vi "ExposeBoundControlValueChangeCallbackVI.vi"(4 "Expose Info":T1, 6 "CtlRef":refnum<vi>, 7 "Event Common Data":cluster{"Source":T2, "Type":T3, "Time":u32} {"Source" items=["LabVIEW UI"=0, "ActiveX"=1, "User Event"=25]}) -> ()   [LabVIEW 2017]
uses:
  <vilib>/event_ctls.llb/eventsource.ctl
  <vilib>/event_ctls.llb/lveventtype.ctl
  Core/ExposeInfo.ctl
  C:/Code/CMCryoSysCode/Expose/COM/CSCom/CSCom/bin/Release/CSCom.dll
  COM/CSCom/CSCom/bin/Release/CSCom.dll
  ExposeParameterBindingData.ctl
  ExposeParameterBindingType.ctl
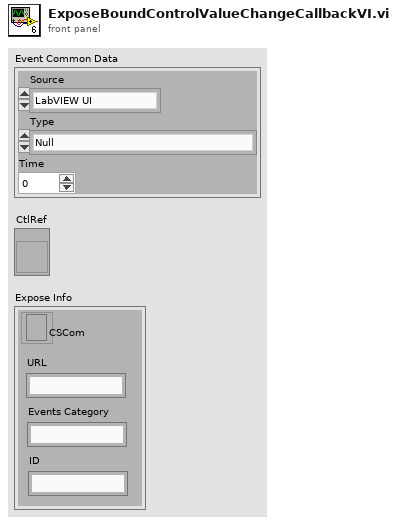
[diagram p1: front panel]
types:
  T1 = typedef "ExposeInfo.ctl" = cluster{"CSCom":refnum<k24>, "URL":string, "Events Category":string, "ID":string}
  T2 = typedef "eventsource.ctl" = u32
  T3 = typedef "lveventtype.ctl" = enum32{"Null", "Timeout", "Annotation Menu Selection", "Annotation Menu Selection?", "App Instance Close", "App Instance Close?", "Autoscale Range Change", "Bookmark Info Change", "Cell Edit", "Cell Edit?", "Cursor Grab", "Cursor Grab?", "Cursor Menu Selection", "Cursor Menu Selection?", "Cursor Move", "Cursor Release", "Data Change", "Direction Change", "Display State Change", "Drag Ended", "Drag Enter", "Drag Leave", "Drag Over", "Drag Source Update", "Drag Starting", "Drag Starting?", "Drop", "Exec State Change", "Key Down", "Key Down?", "Key Repeat", "Key Repeat?", "Key Up", "Listbox Double Click", "Menu Activation?", "Menu Selection (App)", "Menu Selection? (App)", "Menu Selection (User)", "Mouse Down", "Mouse Down?", "Mouse Enter", "Mouse Leave", "Mouse Move", "Mouse Up", "Mouse Wheel", "NI Security User Change (App)", "Pane Size", "Panel Close", "Panel Close?", "Panel Resize", "Plot Attribute Change", "Scale Range Change", "Shortcut Menu Activation?", "Shortcut Menu Selection (App)", "Shortcut Menu Selection? (App)", "Shortcut Menu Selection (User)", "Tree Double Click", "Tree Drag", "Tree Drag?", "Tree Drop", "Tree Drop?", "Tree Item Close", "Tree Item Close?", "Tree Item Open", "Tree Item Open?", "User Event", "Value Change"}
  T4 = typedef "ExposeDataType.ctl" = cluster{"Values":variant, "ParameterBindingInfo":variant}
  T5 = typedef "ExposeParameterBindingData.ctl" = cluster{"Val Change EV":refnum<k27>, "Bind Direction":T6, "Ignore Next\nUpdate Count":i32}
  T6 = typedef "ExposeParameterBindingType.ctl" = enum16{"ToRemote", "FromRemote", "Bidrectional"}
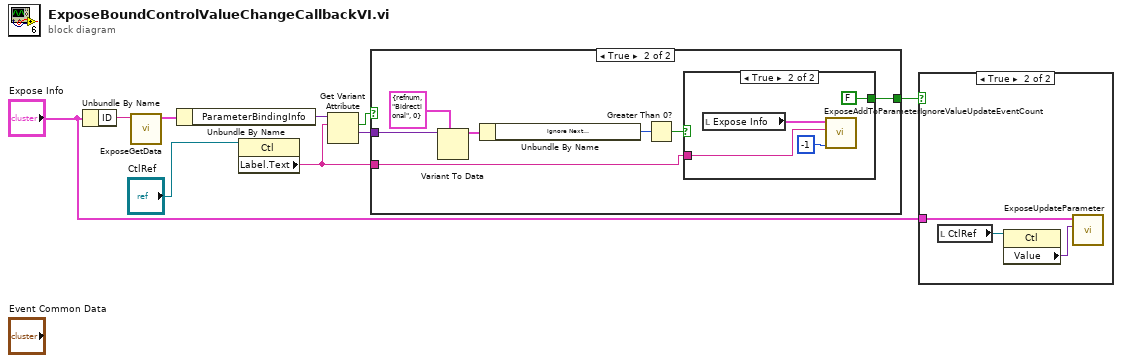
[diagram p0: block diagram]
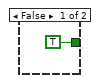
[diagram p3: hidden frame]
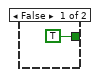
[diagram p4: hidden frame]
diagram:
  n1 = Unbundle By Name("Expose Info") -> ("ID"=w7:string)
  n2 = call "ExposeGetData.vi"("ExposeID"=w7) -> ("ExposeDataType"=w6:T4)  [unwired: 9 in, 1 out]
  n3 = Unbundle By Name(w6) -> ("ParameterBindingInfo"=w5:variant)
  n4 = property class="Ctl"(reference="CtlRef") -> ("Label.Text"=w2:string)  [unwired: 1 in, 2 out]
  n5 = Get Variant Attribute(Variant=w5, name=w2) -> (found=w4:bool, value=w1:variant)  [unwired: 2 in, 2 out]
  n6 = case shown="True" w4 {
    tunnel: [TRUE w13] -> w3
    tunnel: w2 -> [_ w12]
    tunnel: w1 -> [_ w11]
    frame False {
    }
    frame True {
      n7 = Variant To Data(type=T5 {"Val Change EV"=refnum, "Bind Direction"=enum."Bidrectional", "Ignore Next\nUpdate Count"=0} ("ExposeParmeterBindingData"), Variant=w11) -> (data=w16:T5)  [unwired: 1 in, 1 out]
      n8 = Unbundle By Name(w16) -> ("Ignore Next\nUpdate Count"=w15:i32)
      n9 = Greater Than 0?(x=w15) -> (x > 0?=w14:bool)
      n10 = case shown="True" w14 {
        tunnel: [TRUE FALSE] -> w13
        tunnel: w12 -> [_ w20]
        frame False {
        }
        frame True {
          n11 = local read "Expose Info"() -> (w21:T1)
          n12 = call "ExposeAddToParameterIgnoreValueUpdateEventCount.vi"("Add to count (0)"=-1, "Name"=w20, "Expose Info"=w21) -> ()  [unwired: 8 in, 1 out]
        }
      }
    }
  }
  n13 = case shown="True" w3 {
    tunnel: "Expose Info" -> [_ w25]
    frame False {
    }
    frame True {
      n14 = local read "CtlRef"() -> (w24:refnum<vi>)
      n15 = property class="Ctl"(reference=w24) -> ("Value"=w23:variant)  [unwired: 1 in, 2 out]
      n16 = call "ExposeUpdateParameter.vi"("Parameter"=w23, "Expose Info"=w25) -> ()  [unwired: 10 in]
    }
  }
